vi "Write memory hierarchy.vi"(8 "error in (no error)":errorcluster, 10 "memory hierarchy":T1, 11 "NISE_CEF_HierarchyRepo in":refnum<class "NISE_CEF_HierarchyRepo.lvclass">) -> (0 "error out":errorcluster, 3 "NISE_CEF_HierarchyRepo out":refnum<class "NISE_CEF_HierarchyRepo.lvclass">)   [LabVIEW 2014, in "NISE_CEF_HierarchyRepo.lvclass"]
uses:
  NISE_CEF_HierarchyRepo.lvclass
  tree serializer/memory hierarchy.ctl
  tree serializer/full hierarchy.ctl
  tree serializer/hierarchy element.ctl
  serializable configuration/NISE_CEF_serializable configuration.lvclass
  NISE_CEF_HierarchyRepo.lvclass/NISE_CEF_HierarchyRepo.ctl
  tree serializer/NISE_CEF_TreeSerializer.lvlib
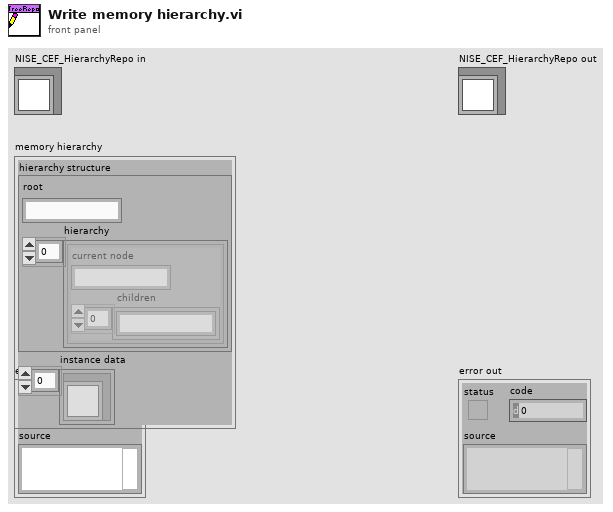
[diagram p1: front panel]
types:
  T1 = typedef "NISE_CEF_TreeSerializer.lvlib/memory hierarchy.ctl" = cluster{"hierarchy structure":T2, "instance data":refnum<class "NISE_CEF_serializable configuration.lvclass">[]}
  T2 = typedef "NISE_CEF_TreeSerializer.lvlib/full hierarchy.ctl" = cluster{"root":string, "hierarchy":T3[]}
  T3 = typedef "NISE_CEF_TreeSerializer.lvlib/hierarchy element.ctl" = cluster{"current node":string, "children":string[]}
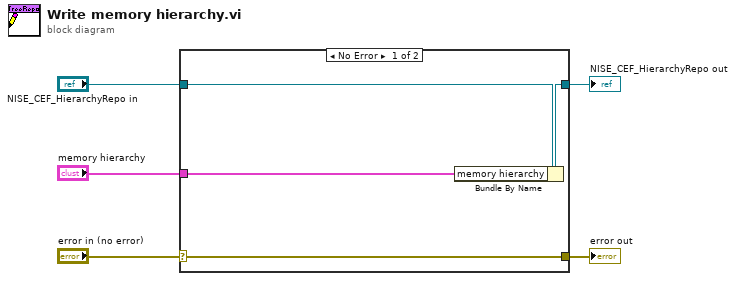
[diagram p0: block diagram]
diagram:
  n1 = case shown="No Error" "error in (no error)" {
    selector: "error in (no error)" -> [w9 w10]
    tunnel: [w9 w10] -> w4
    tunnel: [w7 w11] -> w2
    tunnel: "NISE_CEF_HierarchyRepo in" -> [w8 w11]
    tunnel: "memory hierarchy" -> [w6 _]
    frame No Error {
      n2 = Bundle By Name(cluster=w8, "memory hierarchy"=w6) -> (w7:refnum<class "NISE_CEF_HierarchyRepo.lvclass">)
    }
    frame Error {
    }
  }
  "error out" <- w4
  "NISE_CEF_HierarchyRepo out" <- w2
